vi "tanquemezcla.vi"() -> ()   [LabVIEW 2023]
uses:
  <vilib>/Simulation/ContinuousLinear/Implementation/NILVSim Transfer Function.llb/SIM Transfer Function (SISO).vi
  <vilib>/Simulation/Implementation/XNodeFramework/SimXNode/SimX.xnode
  <vilib>/Simulation/SignalDisplay/Implementation/NILVSim Time Waveform.llb/SIM Time Waveform (scalar).vi
  <vilib>/Simulation/Implementation/Shared/SIMSCR Execution Mode.ctl
  <vilib>/Simulation/Scripting/Companion Diagram/SimConfigNode/_simSolvers.ctl
  <vilib>/Simulation/Scripting/Companion Diagram/SimConfigNode/SimParams.ctl
  <vilib>/Simulation/Scripting/Companion Diagram/SimConfigNode/SimDog.xnode
  <vilib>/Simulation/DataSources/Implementation/NILVSim Step.llb/SIM Step (scalar).vi
panel:
  out "Kvc [m^3·s^(-1)/%]":dbl
  out "Te [C] 2":dbl
  out "Temp":dbl(graph)
  out "Level":dbl(graph)
  in  "?":bool
  in  "Tab Control":T1(tab)
  in  "Valvulas":T2={"Kvs [m^(7/2)·kg^(-1/2)]"=0.00025, "Kvc [m^3·s^(-1)/%]"=3.5e-06}
  in  "Params":T3={"A [m^2]"=1.25, "rho [kg·m^(-3)]"=1500.0, "Cp [Jkg^-1C^1]"=5.0, "Ht [m]"=2.0, "Qe [m3 s^−1] "=0.015, "Tc [C]"=90.0, "Te [C] 2"=25.0, "g"=9.8, "Hi [m] 2"=1.0} {"A [m^2]" format="%.2g"}
  in  "Cluster":T4={"Kt [%·m^(-1)]"=1.0, "KL [%·m^(-1)] "=50.0} {"KL [%·m^(-1)]" min=0.0 max=100.0 step=0.5; "Kt [%·m^(-1)]" min=0.0 max=100.0 step=0.5}
  in  "Inputs":cluster{"u(t) [%]":dbl, "Xvs(t) ":dbl}={"u(t) [%]"=50.0, "Xvs(t) "=0.8} {"Xvs(t)" min=0.0 max=1.0 step=0.01 format="%_2g"; "u(t) [%]" min=0.0 max=100.0 format="%.2g"}
  in  "Simualtion":cluster{"Ts":dbl, "Speed ":dbl}={"Ts"=1.0, "Speed "=40.0}
  out "Yt-Static Characteristic":cluster{"U":dbl[], "Yt":dbl[]}(graph)
  out "YL-Static Characteristic":cluster{"U":dbl[], "YL":dbl[]}(graph)
  out "YT":waveform(dbl)(graph)
  out "YL":waveform(dbl)(graph)
  out "Qe":dbl format="%.4g"
  out "y2 2":dbl format="%#.2g"
  out "Tank":dbl(slide) scale=0.0..2.0 scale format="%#.3g"
  out "y2":dbl format="%#.2g"
  out "ut":dbl format="%.2g"
  out "Qc":dbl format="%.4g"
  out "Qs":dbl format="%.4g"
  # "H(t) [m]"
  # "YL"
  # "YT"
  # "LT"
  # "TT"
  # "u(t) [%]"
  # "TV"
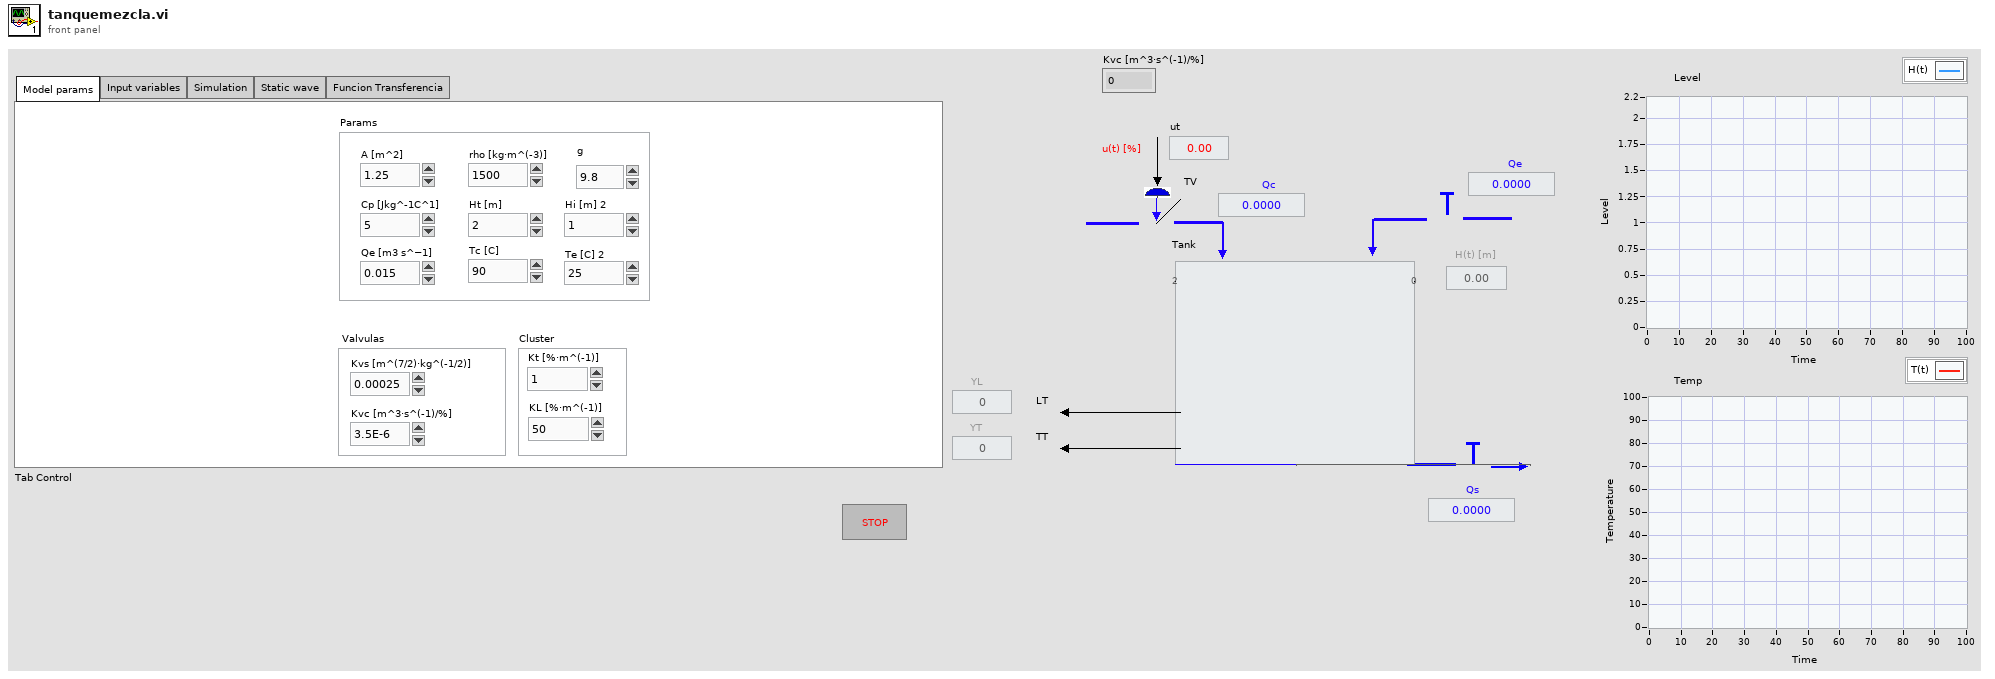
[diagram p1: front panel]
types:
  T1 = enum32{"Model params", "Input variables", "Simulation", "Static wave", "Funcion Transferencia"}
  T2 = cluster{"Kvs [m^(7/2)·kg^(-1/2)]":dbl, "Kvc [m^3·s^(-1)/%]":dbl}
  T3 = cluster{"A [m^2]":dbl, "rho [kg·m^(-3)]":dbl, "Cp [Jkg^-1C^1]":dbl, "Ht [m]":dbl, "Qe [m3 s^−1] ":dbl, "Tc [C]":dbl, "Te [C] 2":dbl, "g":dbl, "Hi [m] 2":dbl}
  T4 = cluster{"Kt [%·m^(-1)]":dbl, "KL [%·m^(-1)] ":dbl}
  T5 = typedef "SimParams.ctl" = cluster{"Initial Time (s)":dbl, "Final Time (s)":dbl, "Step Size (s)":dbl, "ODE Solver":T6, "Minimum Step Size (s)":dbl, "Maximum Step Size (s)":dbl, "Relative Tolerance":dbl, "Absolute Tolerance":dbl, "Software Timing":bool, "Initial Step Size (s)":dbl, "Automatic Fixed Step Size?":bool, "Automatic Discrete Step Size?":bool, "Discrete Step Size (s)":dbl, "Calculate using Time Step":bool, "Solver Wired?":bool, "Prev.Frm.Expected End":u64, "Prev.Frm.Actual End":u64, "Prev.Frm.Finished Late?":bool, "Prev.Iter.Expected End":u64, "Prev.Iter.Actual End":u64, "Prev.Iter.Finished Late?":bool, "Expected Iteration Start":u64, "Actual Iteration Start":u64, "Expected Frame Start":u64, "Actual Frame Start":u64, "Source Name":string, "Name":string, "Period":i64, "Deadline":i64, "Offset":i64, "Start":i64, "Priority":i32, "Timeout":i32, "Processor":i32, "Mode":enum32{"No Change", "Process missed periods, maintain original phase", "Discard missed periods, maintain original phase", "Process missed periods, ignore original phase", "Discard missed periods, ignore original phase"}, "Wakeup reason":enum32{"Normal", "Aborted", "Asynchronous wakeup", "Timing source error", "Timed loop error", "Timeout"}, "Error":errorcluster, "Source Type":string, "Secondary Source Type":string, "Global End Time":u64, "Global Start Time":u64, "Full Solver Reset":bool, "Execution Mode":T7, "Nan/Inf Check":bool, "Custom Solver Library":string, "Solver Is Variable":bool, "custom solver name":string, "Signal Collection Decimation":u32}
  T6 = typedef "_simSolvers.ctl" = enum16{"Runge-Kutta 1 (Euler)", "Runge-Kutta 2", "Runge-Kutta 3", "Runge-Kutta 4", "Runge-Kutta 23 (variable)", "Runge-Kutta 45 (variable)", "BDF (variable)", "Adams-Moulton (variable)", "Rosenbrock (variable)", "Discrete States Only", "SDIRK 4 (variable)", "Radau 5 (variable)", "Radau 9 (variable)", "Radau 13 (variable)", "Radau [Variable Order] (variable)", "Gear's Method (variable)", "Linearizer", "State Query", "Trim Eval", "Custom Solver"}
  T7 = typedef "SIMSCR Execution Mode.ctl" = enum16{"Simulate to Completion", "Single Time-Step Simulation (Fixed Step Only)"}
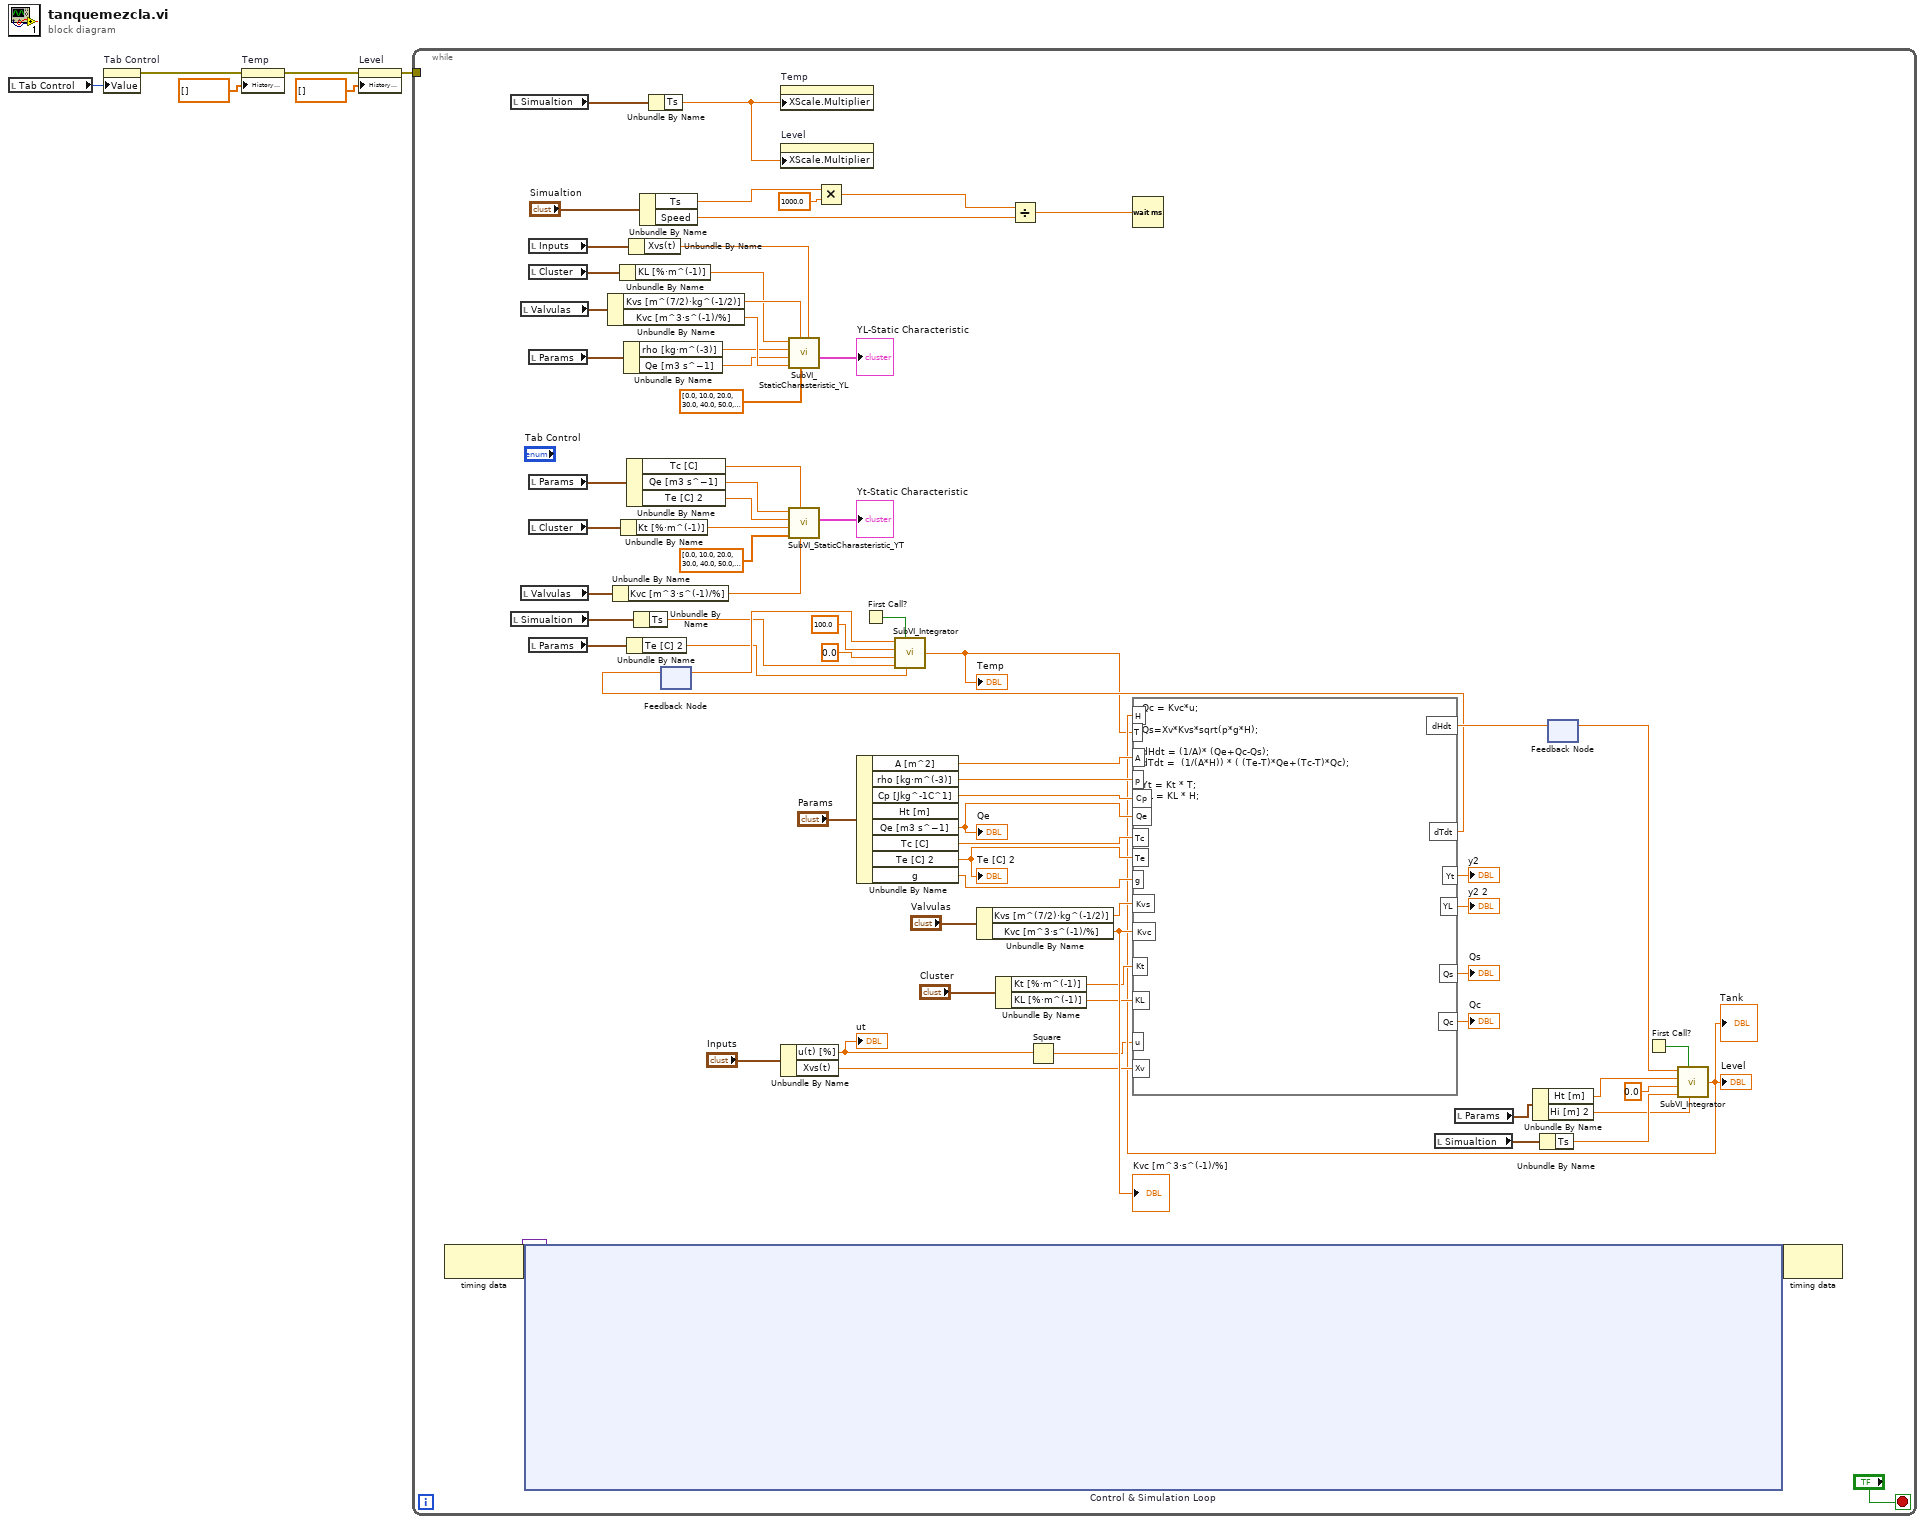
[diagram p0: block diagram]
diagram:
  n1 = local read "Tab Control"() -> (w6:T1)
  n2 = property on="Tab Control" class="TabCtl (strict)"("Value"=w6) -> (error out=w5:errorcluster)  [unwired: 2 in, 1 out]
  n3 = property on="Temp" class="WFChart (strict)"(error in=w5, "History Data"=dbl[] []) -> (error out=w4:errorcluster)  [unwired: 1 in, 1 out]
  n4 = property on="Level" class="WFChart (strict)"(error in=w4, "History Data"=dbl[] []) -> (error out=w3:errorcluster)  [unwired: 1 in, 1 out]
  n5 = while {
    tunnel: w3 -> [_]
    stop <- "?" stop-if-true
    n6 = node-c288() -> (w8:variant)  [unwired: 1 in]
    n7 = local read "Simualtion"() -> (w35:cluster{"Ts":dbl, "Speed ":dbl})
    n8 = local read "Simualtion"() -> (w46:cluster{"Ts":dbl, "Speed ":dbl})
    n9 = local read "Valvulas"() -> (w17:T2)
    n10 = local read "Valvulas"() -> (w23:T2)
    n11 = node-c254 "Control & Simulation Loop"(w8) -> (w7:variant)
    n12 = local read "Inputs"() -> (w19:cluster{"u(t) [%]":dbl, "Xvs(t) ":dbl})
    n13 = local read "Cluster"() -> (w15:T4)
    n14 = local read "Params"() -> (w11:T3)
    n15 = local read "Params"() -> (w30:T3)
    n16 = local read "Cluster"() -> (w26:T4)
    n17 = local read "Params"() -> (w42:T3)
    n18 = Unbundle By Name(w17) -> ("Kvs [m^(7/2)·kg^(-1/2)]"=w16:dbl, "Kvc [m^3·s^(-1)/%]"=w13:dbl)
    n19 = Unbundle By Name(w23) -> ("Kvc [m^3·s^(-1)/%]"=w22:dbl)
    n20 = Unbundle By Name(w15) -> ("KL [%·m^(-1)]"=w14:dbl)
    n21 = Unbundle By Name(w26) -> ("Kt [%·m^(-1)]"=w25:dbl)
    n22 = Unbundle By Name(w11) -> ("rho [kg·m^(-3)]"=w10:dbl, "Qe [m3 s^−1]"=w9:dbl)
    n23 = Unbundle By Name(w30) -> ("Tc [C]"=w29:dbl, "Qe [m3 s^−1]"=w28:dbl, "Te [C] 2"=w27:dbl)
    n24 = Unbundle By Name(w42) -> ("Te [C] 2"=w41:dbl)
    n25 = Unbundle By Name(w19) -> ("Xvs(t)"=w18:dbl)
    n26 = Unbundle By Name(w46) -> ("Ts"=w45:dbl)
    n27 = Unbundle By Name("Simualtion") -> ("Ts"=w58:dbl, "Speed"=w57:dbl)
    n28 = Unbundle By Name(w35) -> ("Ts"=w34:dbl)
    n29 = feedback #1() -> (w47:dbl)  [unwired: 1 in]
    n30 = property on="Temp" class="WFChart (strict)"("XScale.Multiplier"=w34) -> ()  [unwired: 2 in, 2 out]
    n31 = property on="Level" class="WFChart (strict)"("XScale.Multiplier"=w34) -> ()  [unwired: 2 in, 2 out]
    n32 = Unbundle By Name("Inputs") -> ("u(t) [%]"=w32:dbl, "Xvs(t)"=w68:dbl)
    "ut" <- w32
    n33 = call "SubVI_StaticCharasteristic_YL.vi"("Xs"=w18, "U"=dbl[] [0.0, 10.0, 20.0, 30.0, 40.0, 50.0, 60.0, 70.0, 80.0, 90.0, 100.0], "Kvs"=w16, "Kvc"=w13, "Qe"=w9, "rho"=w10, "KL"=w14) -> ("Cluster"=→"YL-Static Characteristic":cluster{"U":dbl[], "YL":dbl[]})  [unwired: 4 in]
    n34 = call "SubVI_StaticCharasteristic_YT.vi"("Kvc"=w22, "Tc"=w29, "U"=dbl[] [0.0, 10.0, 20.0, 30.0, 40.0, 50.0, 60.0, 70.0, 80.0, 90.0, 100.0], "Kt"=w25, "Te"=w27, "Qe"=w28) -> ("Output"=→"Yt-Static Characteristic":cluster{"U":dbl[], "Yt":dbl[]})  [unwired: 5 in]
    n35 = Multiply(x=w58, y=1000.0) -> (x*y=w61:dbl)
    n36 = Unbundle By Name("Params") -> ("A [m^2]"=w80:dbl, "rho [kg·m^(-3)]"=w79:dbl, "Cp [Jkg^-1C^1]"=w78:dbl, "Qe [m3 s^−1]"=w39:dbl, "Tc [C]"=w77:dbl, "Te [C] 2"=w70:dbl, "g"=w69:dbl)  [unwired: 1 out]
    "Qe" <- w39
    "Te [C] 2" <- w70
    n37 = First Call?() -> (First Call?: T/F=w37:bool)
    n38 = call "SubVI_Integrator.vi"("y_init"=w41, "Init"=w37, "T_step [s]"=w45, "y_min"=0.0, "y_max"=100.0, "u"=w47) -> ("y"=w33:dbl)
    "Temp" <- w33
    n39 = Unbundle By Name("Valvulas") -> ("Kvs [m^(7/2)·kg^(-1/2)]"=w76:dbl, "Kvc [m^3·s^(-1)/%]"=w75:dbl)
    "Kvc [m^3·s^(-1)/%]" <- w75
    n40 = Unbundle By Name("Cluster") -> ("Kt [%·m^(-1)]"=w72:dbl, "KL [%·m^(-1)]"=w71:dbl)
    n41 = Divide(x=w61, y=w57) -> (x/y=w60:dbl)
    n42 = Square(x=w32) -> (x^2=w31:dbl)
    n43 = Wait (ms)(milliseconds to wait=w60) -> ()  [unwired: 1 out]
    n44 = local read "Simualtion"() -> (w56:cluster{"Ts":dbl, "Speed ":dbl})
    n45 = local read "Params"() -> (w51:T3)
    n46 = Unbundle By Name(w51) -> ("Ht [m]"=w50:dbl, "Hi [m] 2"=w49:dbl)
    n47 = Unbundle By Name(w56) -> ("Ts"=w55:dbl)
    n48 = feedback #2() -> (w54:dbl)  [unwired: 1 in]
    n49 = First Call?() -> (First Call?: T/F=w38:bool)
    n50 = call "SubVI_Integrator.vi"("y_init"=w49, "Init"=w38, "T_step [s]"=w55, "y_min"=0.0, "y_max"=w50, "u"=w54) -> ("y"=w36:dbl)
    "Tank" <- w36
    "Level" <- w36
    n51 = formula code="Qc = Kvc*u;\n\nQs=Xv*Kvs*sqrt(p*g*H);\n\ndHdt = (1/A)* (Qe+Qc-Qs);\ndTdt =  (1/(A*H)) * ( (Te-T)*Qe+(Tc-T)*Qc);\n\nYt = Kt * T;\nYL = KL * H;"("A"=w80, "H"=w36, "p"=w79, "g"=w69, "Kvc"=w75, "Kt"=w72, "KL"=w71, "Kvs"=w76, "u"=w31, "Xv"=w68, "Qe"=w39, "Te"=w70, "Tc"=w77, "T"=w33, "Cp"=w78) -> ("Qs"=→"Qs":dbl, "Yt"=→"y2":dbl, "YL"=→"y2 2":dbl, "dHdt"=w53:dbl, "dTdt"=w48:dbl, "Qc"=→"Qc":dbl)
    n52 = feedback-in #1(w48) -> ()
    n53 = feedback-in #2(w53) -> ()
    n54 = node-c288(w7) -> ()  [unwired: 1 out]
  }
